vi "Format Tables with 2 Digit Precision.vi"(0 "Header":string[](array[string]), 5 "Data Table":dbl[][](array[numeric]), 7 "upper limit":dbl, 9 "lower limit":dbl) -> (4 "spreadsheet string":string, 8 "Table Passed?":bool)   [LabVIEW 2010]
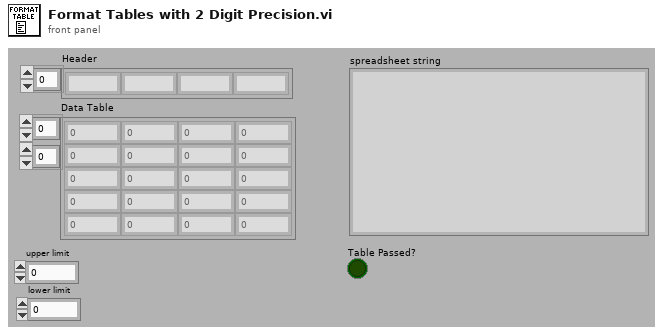
[diagram p1: front panel]
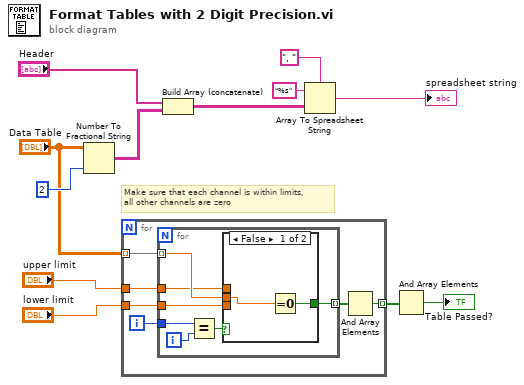
[diagram p0: block diagram]
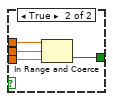
[diagram p2: hidden frame]
diagram:
  # "Make sure that each channel is within limits,\nall other channels are zero"
  n1 = Number To Fractional String(number="Data Table", precision (6)=i16 2) -> (F-format string=w11:string[][])  [unwired: 2 in]
  n2 = for {
    tunnel: "Data Table" -> [w18] mode=indexing
    tunnel: "upper limit" -> [w16]
    tunnel: "lower limit" -> [w15]
    tunnel: [w13] -> w2 mode=indexing
    i -> [w17]
    n3 = for {
      tunnel: w18 -> [w22] mode=indexing
      tunnel: w17 -> [w24]
      tunnel: w16 -> [w21]
      tunnel: w15 -> [w20]
      tunnel: [w19] -> w14 mode=indexing
      i -> [w25]
      n4 = Equal?(x=w24, y=w25) -> (x = y?=w23:bool)
      n5 = case shown="False" w23 {
        tunnel: w22 -> [w26 w31]
        tunnel: w21 -> [_ w30]
        tunnel: w20 -> [_ w29]
        tunnel: [w27 w28] -> w19
        frame False {
          n6 = Equal To 0?(x=w26) -> (x = 0?=w27:bool)
        }
        frame True {
          n7 = In Range and Coerce(upper limit=w30, x=w31, lower limit=w29) -> (In Range?=w28:bool)  [unwired: 1 out]
        }
      }
    }
    n8 = And Array Elements(Boolean array=w14) -> (logical AND=w13:bool)
  }
  n9 = Build Array (concatenate)("Header", w11) -> (w9:string[][])
  n10 = Array To Spreadsheet String(delimiter (Tab)=", ", array=w9, 3:"%s" ("format string")) -> (spreadsheet string=→"spreadsheet string":string)
  n11 = And Array Elements(Boolean array=w2) -> (logical AND=→"Table Passed?":bool)
